vi "KH_DAQ_InitFGlob.vi"(8 "EIP_DO":T1 {"Nr" max=63; "Chan" max=63}, 9 "EIP_DI":T3 {"Nr" max=63; "Chan" max=63}, 10 "EIP_AI":T4 {"Offset" format="%.4f"; "Phys Max" format="%.4f"; "Phys Min" format="%.4f"}, 11 "EIP_AO":T7 {"Offset" format="%.4f"; "Phys Max" format="%.4f"; "Phys Min" format="%.4f"}) -> ()   [LabVIEW 2021]
uses:
  KH_DAQ_TypeDefs_Cluster AO.ctl
  KH_DAQ_TypeDefs_Messbereich.ctl
  KH EthernetIPConfig 17.14/KH EthernetIPConfig TypeDefs ModuleTyp.ctl
  KH_DAQ_TypeDefs_Bereich.ctl
  KH_DAQ_TypeDefs_Cluster AI.ctl
  Turck/KH_DAQ_TURCK_TypeDefs_Cluster DI.ctl
  Turck/KH_DAQ_TURCK_TypeDefs_Cluster DO.ctl
  KH Turck EthernetIP 17.12/KH TURCK TypeDefs FGlob.ctl
  XLP80_ProjectLibs/XLP80_FGlob/1886_FGlob_TDefs_Enum_FGlobItems.ctl
  Turck/KH_DAQ_TURCK_Global.vi
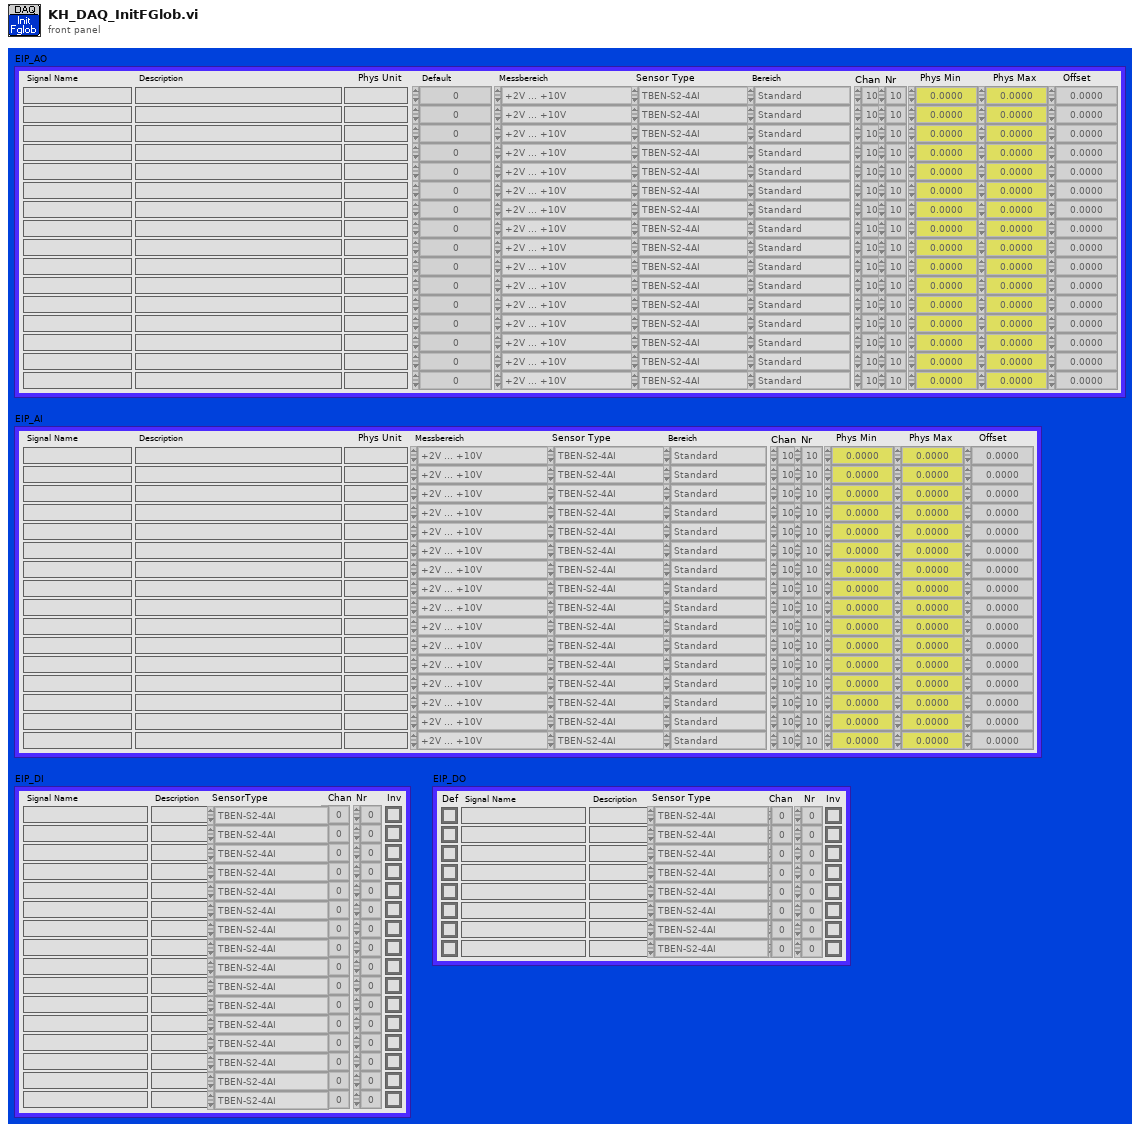
[diagram p1: front panel]
types:
  T1 = typedef "KH_DAQ_TURCK_TypeDefs_Cluster DO.ctl" = cluster{"Def":bool[], "Signal Name":string[], "Description":string[], "Chan":u16[], "Inv":bool[], "Nr":u16[], "SensorType":T2[]}
  T2 = typedef "KH EthernetIPConfig TypeDefs ModuleTyp.ctl" = enum16{"TBEN-S2-4AI", "TBEN-S1-8DXP", "TBEN-S2-2RFID-4DXP", "TBEN-S2-4AO", "TBEN-S2-4IOL"}
  T3 = typedef "KH_DAQ_TURCK_TypeDefs_Cluster DI.ctl" = cluster{"Signal Name":string[], "Description":string[], "Chan":u16[], "Inv":bool[], "Nr":u16[], "SensorType":T2[]}
  T4 = typedef "KH_DAQ_TypeDefs_Cluster AI.ctl" = cluster{"Signal Name":string[], "Description":string[], "Phys Unit":string[], "Messbereich":T5[], "Chan":u16[], "Phys Min":sgl[], "Phys Max":sgl[], "Offset":sgl[], "Nr":u16[], "SensorType 2":T2[], "Bereich":T6[]}
  T5 = typedef "KH_DAQ_TypeDefs_Messbereich.ctl" = enum16{"-10V ... +10V", "0V ... +10V", "+2V ... +10V", "0V ... +5V", "+1V ... +5V", "-1V ... +1V", "-500mV ... +500mV", "-100mV ... +100mV", "-50mV ... +50mV", "0mA ... +20mA", "+4mA ... +20mA", "-20mA ... +20mA", "0 Ohm ... 100 Ohm", "0 Ohm ... 400 Ohm", "0 Ohm ... 2000 Ohm", "0 Ohm ... 4000 Ohm", "-200°C ... 150°C PT100", "-200°C ... 150°C PT200", "-200°C ... 150°C PT500", "-200°C ... 150°C PT1000", "-60°C ... 150°C Ni100", "-60°C ... 150°C Ni1000", "-200°C ... 850°C PT100", "-200°C ... 850°C PT200", "-200°C ... 850°C PT500", "-200°C ... 850°C PT1000", "-50°C ... 250°C Ni100", "-50°C ... 250° Ni 1000"}
  T6 = typedef "KH_DAQ_TypeDefs_Bereich.ctl" = enum16{"Standard", "extended Range", "NE43", ""}
  T7 = typedef "KH_DAQ_TypeDefs_Cluster AO.ctl" = cluster{"Signal Name":string[], "Description":string[], "Phys Unit":string[], "Messbereich":T5[], "Chan":u16[], "Phys Min":sgl[], "Phys Max":sgl[], "Offset":sgl[], "Nr":u16[], "SensorType 2":T2[], "Bereich":T6[], "Default":sgl[]}
  T8 = typedef "1886_FGlob_TDefs_Enum_FGlobItems.ctl" = enum16{"Put one", "Put all", "Recall one", "Recall all"}
  T9 = typedef "KH TURCK TypeDefs FGlob.ctl" = enum16{"Put one", "Put all", "Recall one", "Recall all"}
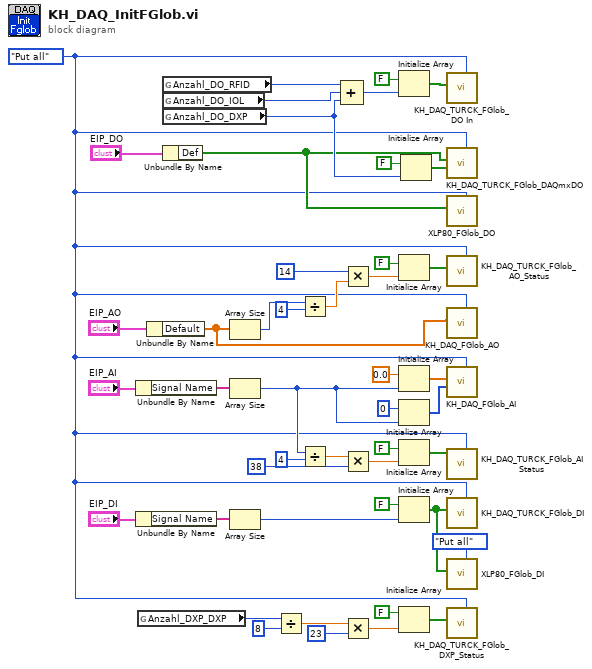
[diagram p0: block diagram]
diagram:
  w2 = KH_TURCK_TypeDefs_FGlob."Put all" ("Function")
  n1 = Unbundle By Name("EIP_AI") -> ("Signal Name"=w40:string[])
  n2 = Unbundle By Name("EIP_DI") -> ("Signal Name"=w26:string[])
  n3 = global read "KH_DAQ_TURCK_Global.vi" "Anzahl_DXP_DXP"() -> (w8:i32)
  n4 = Unbundle By Name("EIP_AO") -> ("Default"=w6:sgl[])
  n5 = global read "KH_DAQ_TURCK_Global.vi" "Anzahl_DO_RFID"() -> (w44:i32)
  n6 = global read "KH_DAQ_TURCK_Global.vi" "Anzahl_DO_IOL"() -> (w45:i32)
  n7 = global read "KH_DAQ_TURCK_Global.vi" "Anzahl_DO_DXP"() -> (w16:i32)
  n8 = Unbundle By Name("EIP_DO") -> ("Def"=w3:bool[])
  n9 = Array Size(array=w6) -> (size(s)=w14:i32)
  n10 = Array Size(array=w40) -> (size(s)=w11:i32)
  n11 = Array Size(array=w26) -> (size(s)=w19:i32)
  n12 = Divide(x=w8, y=8) -> (x/y=w7:dbl)
  n13 = Divide(x=w14, y=4) -> (x/y=w13:sgl)
  n14 = Divide(x=w11, y=4) -> (x/y=w10:sgl)
  n15 = Compound Arithmetic op=ADD(w44, w45, w16) -> (w46:i32)
  n16 = Multiply(x=14, y=w13) -> (x*y=w32:sgl)
  n17 = Multiply(x=w10, y=38 ("x")) -> (x*y=w30:sgl)
  n18 = Multiply(x=w7, y=23 ("x")) -> (x*y=w22:dbl)
  n19 = Initialize Array(FALSE ("values"), w46) -> (w41:bool[])
  n20 = Initialize Array(FALSE, w32) -> (w33:bool[])
  n21 = Initialize Array(sgl 0.0 ("values"), w11) -> (w36:sgl[])
  n22 = Initialize Array(i16 0 ("element"), w11) -> (w35:i16[])
  n23 = Initialize Array(FALSE, w30) -> (w28:bool[])
  n24 = Initialize Array(FALSE, w19) -> (w4:bool[])
  n25 = Initialize Array(FALSE, w22) -> (w21:bool[])
  n26 = Initialize Array(FALSE ("values"), w16) -> (w17:bool[])
  n27 = call "KH_DAQ_TURCK_FGlob_DO In.vi"("Function (Recall One)"=w2, "DO in Values IN"=w41) -> ()  [unwired: 7 in, 3 out]
  n28 = call "KH_DAQ_TURCK_FGlob_DAQmxDO.vi"("Function (Recall One)"=w2, "DXP Reset IN"=w17, "DXP Values IN"=w3) -> ()  [unwired: 5 in, 4 out]
  n29 = call "XLP80_FGlob_DO.vi"("Function (Set)"=w2, "DXP Values IN"=w3) -> ()  [unwired: 7 in, 3 out]
  n30 = call "KH_DAQ_TURCK_FGlob_AO_Status.vi"("Function (Recall One)"=w2, "AO Status IN"=w33) -> ()  [unwired: 8 in, 2 out]
  n31 = call "KH_DAQ_FGlob_AO.vi"("Function (Recall One)"=w2, "AO Values IN"=w6) -> ()  [unwired: 7 in, 3 out]
  n32 = call "KH_DAQ_FGlob_AI.vi"("Function (Recall One)"=w2, "AI Unscaled IN"=w35, "AI Values IN"=w36) -> ()  [unwired: 5 in, 4 out]
  n33 = call "KH_DAQ_TURCK_FGlob_AI Status.vi"("Function (Recall One)"=w2, "StatusIn"=w28) -> ()  [unwired: 7 in, 3 out]
  n34 = call "KH_DAQ_TURCK_FGlob_DI.vi"("Function (Recall One)"=w2, "DI Values IN"=w4) -> ()  [unwired: 7 in, 3 out]
  n35 = call "XLP80_FGlob_DI.vi"("Function (Recall One)"=1886_FGlob_TDefs_Enum_FGlobItems."Put all", "DI Values IN"=w4) -> ()  [unwired: 7 in, 3 out]
  n36 = call "KH_DAQ_TURCK_FGlob_DXP_Status.vi"("Function (Recall One)"=w2, "DXP Status IN"=w21) -> ()  [unwired: 8 in, 2 out]
